vi "Calibration_Hall.vi"(0 "Dwell Time (ms)":u32, 1 "R array in (V)":dbl[](array[numeric]), 2 "Max Field":dbl=0.5 format="%#_13g", 3 "Reset Field":dbl, 4 "B array in (T)":dbl[](array[numeric]), 5 "Set Field (T)":dbl=0.3, 7 "dB":dbl) -> (10 "R array out (V)":dbl[](array[numeric]), 11 "Ready?":bool, 14 "Calibration Curve":dbl[][](array[numeric]), 15 "Calibration Curve":cluster{dbl[], dbl[]}[](graph), 16 "B array Out":dbl[](array[numeric]), 19 "Set Field out":dbl)   [LabVIEW 2015]
uses:
  oxford_driver/Oxford Drivers/BUSGEN.LLB/OxfordAddress.ctl
panel:
  # "a0+a1*x+a2*x^2+a3*x^3+a4*x^4+a5*x^5"
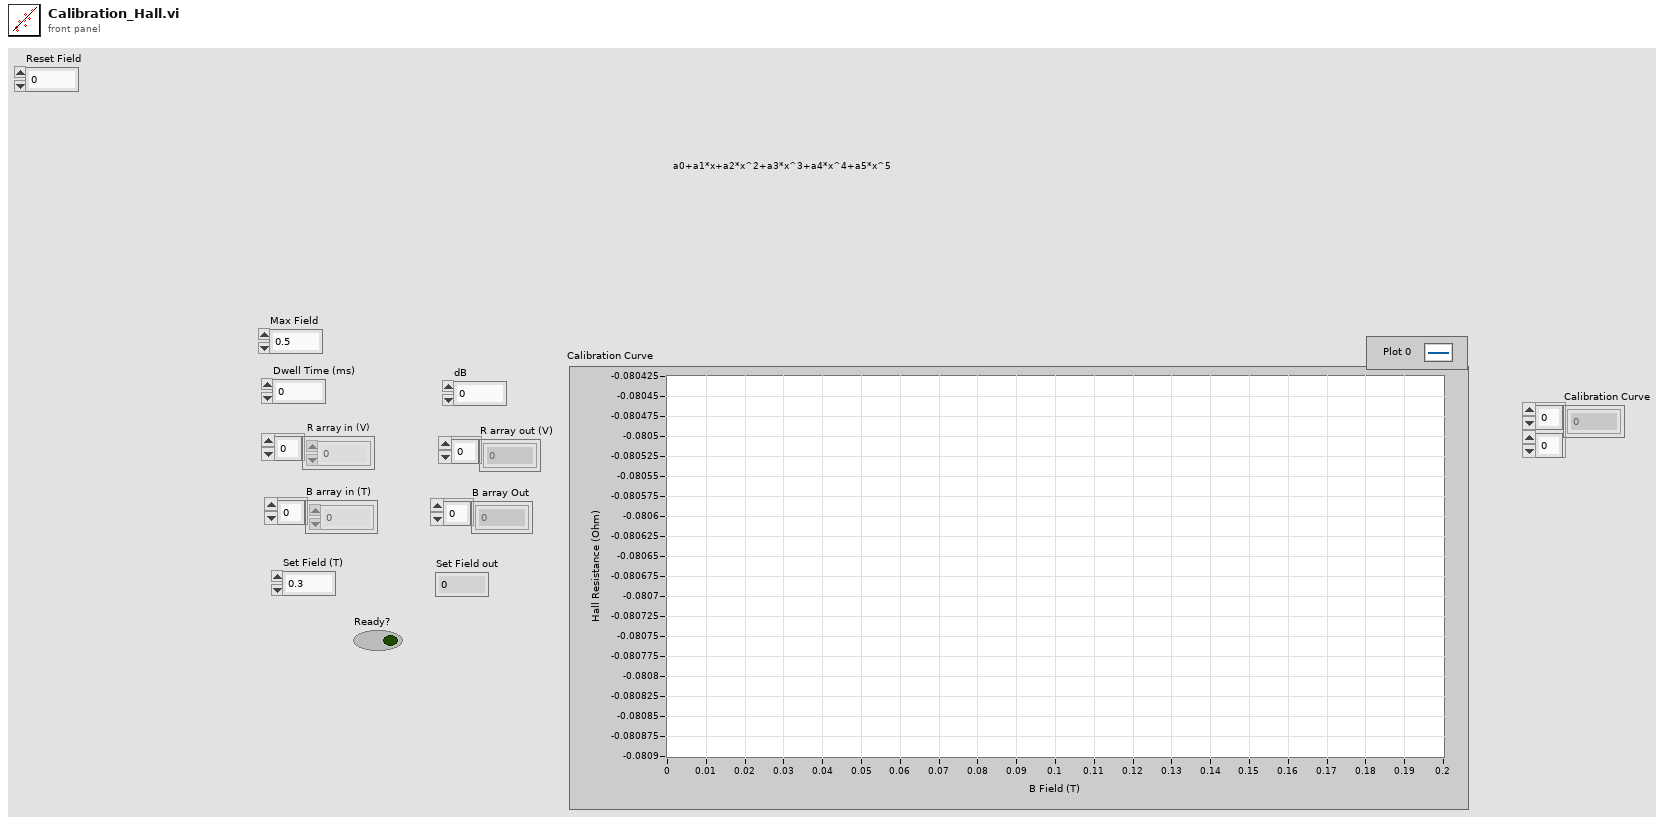
[diagram p1: front panel]
types:
  T1 = typedef "OxfordAddress.ctl" = cluster{"Com Port":i32, "ISOBUS Address":i32, "GPIB Address":i16, "Communication":enum16{"RS232", "ISOBUS", "GPIB", "Gateway"}}
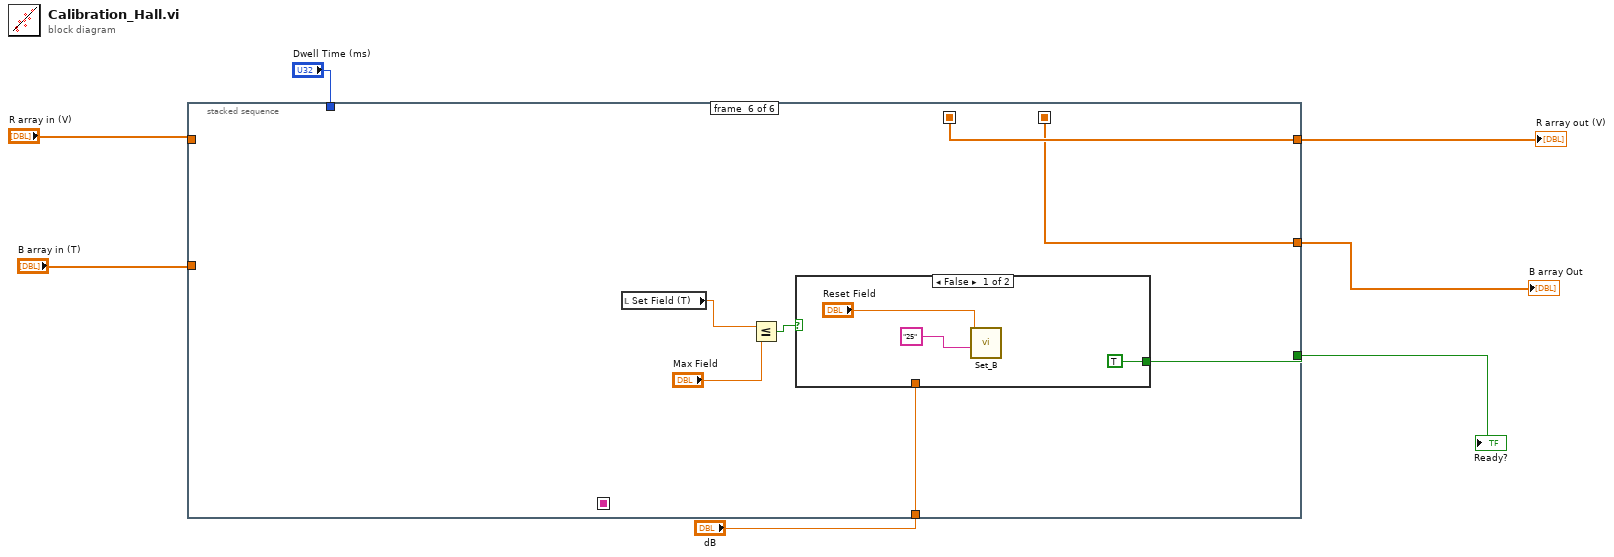
[diagram p0: block diagram]
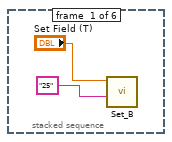
[diagram p2: hidden frame]
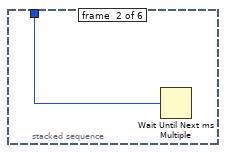
[diagram p3: hidden frame]
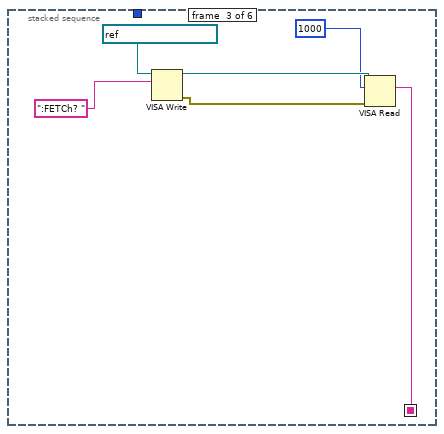
[diagram p4: hidden frame]
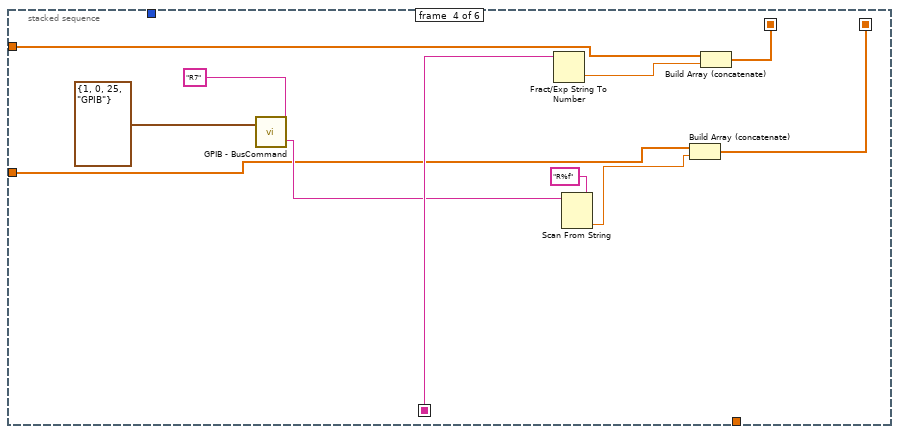
[diagram p5: hidden frame]
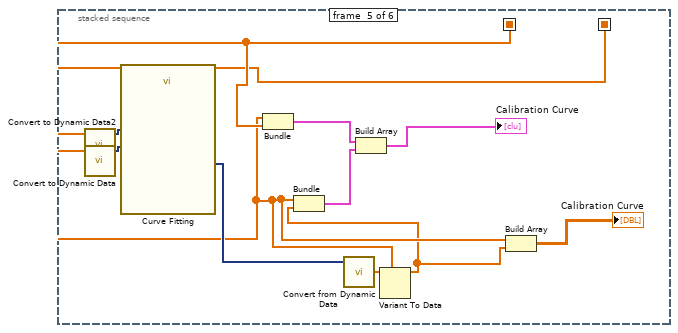
[diagram p6: hidden frame]
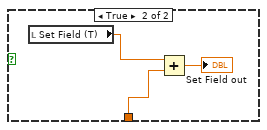
[diagram p7: hidden frame]
diagram:
  n1 = stacked-sequence {
    seq-local: [_ _ w11 _ _ _] -> [_ _ _ w24 _ _]
    seq-local: [_ _ _ w18 _ _] -> [_ _ _ _ w31 w40]
    seq-local: [_ _ _ w17 _ _] -> [_ _ _ _ w30 w39]
    tunnel: [_ _ _ _ _ w43] -> w3
    tunnel: [_ _ _ _ _ w40] -> w2
    tunnel: "R array in (V)" -> [_ _ _ w22 _ _]
    tunnel: [_ _ _ _ _ w39] -> w1
    tunnel: "B array in (T)" -> [_ _ _ w20 _ _]
    tunnel: "dB" -> [_ _ _ _ _ w42]
    tunnel: "Dwell Time (ms)" -> [_ w10 _ _ _ _]
    frame #0 {
      n2 = call "Set_B.vi"("address string"="25", "Set Field (T)"="Set Field (T)") -> ()  [unwired: 9 in, 1 out]
    }
    frame #1 {
      n3 = Wait Until Next ms Multiple(millisecond multiple=w10) -> ()  [unwired: 1 out]
    }
    frame #2 {
      n4 = VISA Write(VISA resource name=refnum<visa-resource-name> "GPIB0::19::INSTR", write buffer=":FETCh? " ("data")) -> (VISA resource name out=w16:refnum<visa-resource-name>, error out=w12:errorcluster)  [unwired: 1 in, 1 out]
      n5 = VISA Read(VISA resource name=w16, byte count=u32 1000, error in (no error)=w12) -> (read buffer=w11:string)  [unwired: 3 out]
    }
    frame #3 {
      n6 = call "GPIB - BusCommand.vi"("Command"="R7" ("write buffer"), "Address"=T1 {"Com Port"=1, "ISOBUS Address"=0, "GPIB Address"=25, "Communication"=enum."GPIB"}) -> ("Reply"=w23:string)  [unwired: 1 out]
      n7 = Fract/Exp String To Number(string=w24) -> (number=w19:dbl)  [unwired: 3 in, 1 out]
      n8 = Scan From String(format string="R%f" ("remaining string"), input string=w23) -> (output 1=w21:dbl)  [unwired: 3 in, 3 out]
      n9 = Build Array (concatenate)(w20, w21) -> (w17:dbl[])
      n10 = Build Array (concatenate)(w22, w19) -> (w18:dbl[])
    }
    frame #4 {
      n11 = call "Convert to Dynamic Data2"("Array"=w31) -> ("Dynamic Data Type"=w37:dynamicdata)  [unwired: 3 in]
      n12 = call "Convert to Dynamic Data"("Array"=w30) -> ("Dynamic Data Type"=w38:dynamicdata)  [unwired: 3 in]
      n13 = call "Curve Fitting"("Locations"=w38, "Signals"=w37) -> ("best fit"=w35:dynamicdata)  [unwired: 6 in, 3 out]
      n14 = Bundle(w30, w31) -> (w36:cluster{dbl[], dbl[]})  [unwired: 1 in]
      n15 = call "Convert from Dynamic Data"("Dynamic Data Type"=w35) -> ("Array"=w34:dbl[])  [unwired: 3 in]
      n16 = Variant To Data(type=w30, Variant=w34) -> (data=w29:dbl[])  [unwired: 1 in, 1 out]
      n17 = Bundle(w30, w29) -> (w33:cluster{dbl[], dbl[]})  [unwired: 1 in]
      n18 = Build Array(w36, w33) -> (→"Calibration Curve":cluster{dbl[], dbl[]}[])
      n19 = Build Array(w30, w29) -> (→"Calibration Curve":dbl[][])
    }
    frame #5 {
      n20 = local read "Set Field (T)"() -> (w41:dbl)
      n21 = Less Or Equal?(x=w41, y="Max Field") -> (x <= y?=w45:bool)
      n22 = case shown="False" w45 {
        tunnel: [TRUE _] -> w43
        tunnel: w42 -> [_ w51]
        frame False {
          n23 = call "Set_B.vi"("address string"="25", "Set Field (T)"="Reset Field") -> ()  [unwired: 9 in, 1 out]
        }
        frame True {
          n24 = local read "Set Field (T)"() -> (w50:dbl)
          n25 = Add(x=w50, y=w51) -> (x+y=→"Set Field out":dbl)
        }
      }
    }
  }
  "R array out (V)" <- w2
  "B array Out" <- w1
  "Ready?" <- w3
